vi "Handle Camera Configuration.vi"(9 "CameraNameRef":refnum<vi>, 10 "Camera File Name":string="Camera", 11 "ClusterRef":refnum<vi>) -> ()   [LabVIEW 2016]
uses:
  <vilib>/Rock Robotics/Network Tables/Make Table Operation.ctl
  <vilib>/Utility/config.llb/Read Key (String).vi
  <vilib>/Utility/config.llb/Read Key (I32).vi
  <vilib>/Utility/config.llb/Write Key (String).vi
  <vilib>/Utility/config.llb/Write Key (I32).vi
  <vilib>/Utility/config.llb/NI_LVConfig.lvlib
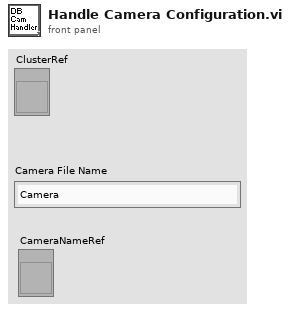
[diagram p1: front panel]
types:
  T1 = typedef "NI_LVConfig.lvlib/Config Data RefNum.ctl" = refnum<k1>
  T2 = cluster{"value":i32, "value":i32, "index":i32, bool}
  T3 = typedef "Make Table Operation.ctl" = enum16{"Get or Add Field", "Get Field or Add Temp", "Replace Temp ID", "Get Field ID - No Add", "Get Table Field IDs", "Get Field ID Info", "Move Field to Temp", "Validate", "Remove Field", "Remove All"}
  T4 = cluster{"Frame Rate":i32, "Compression":i32, "Size":u16, "DB Camera Config":bool}
  T5 = typedef "Field ID.ctl" = i32
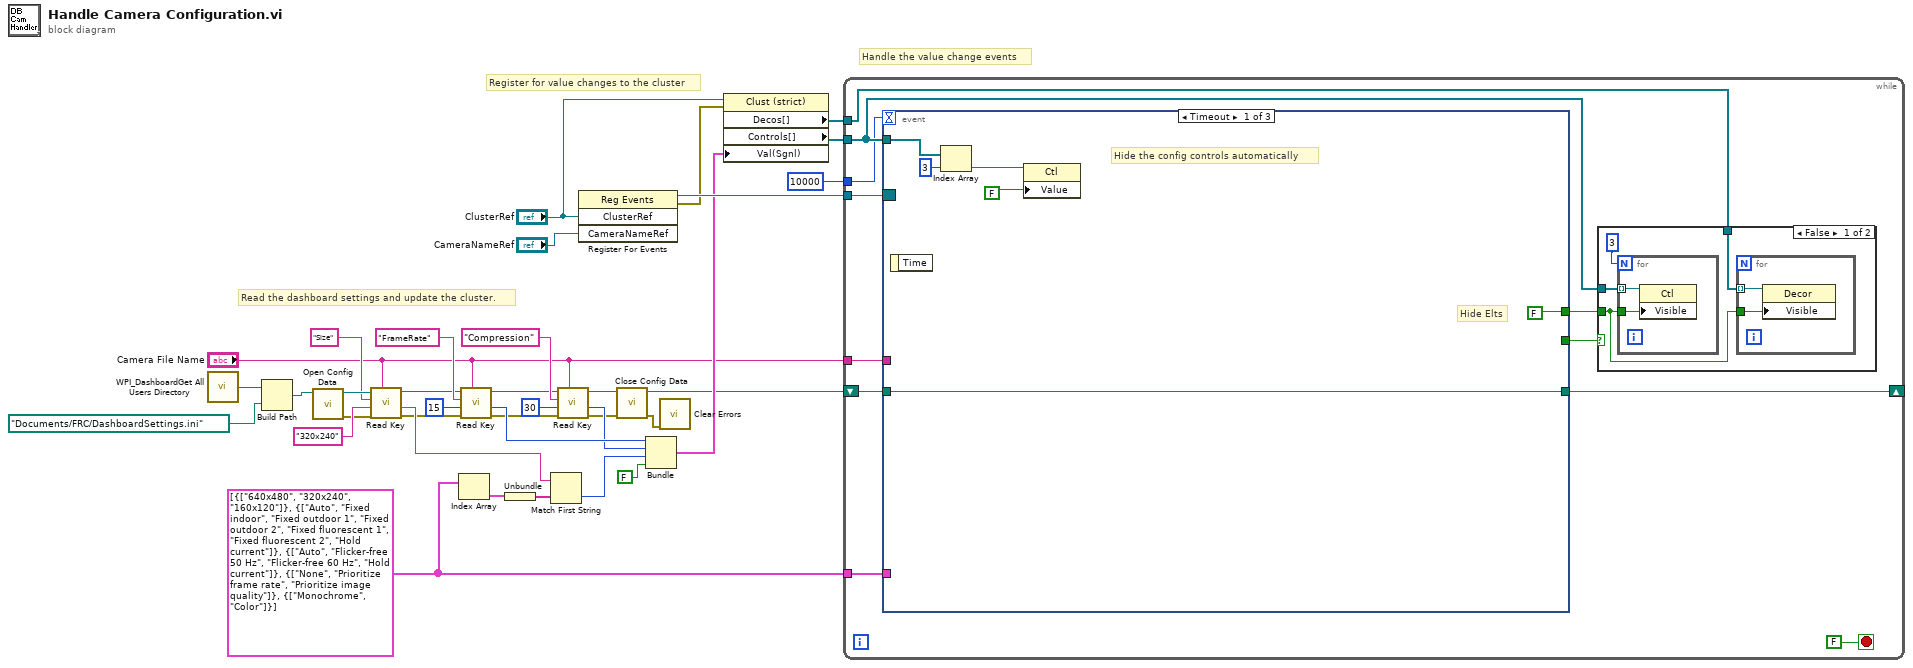
[diagram p0: block diagram]
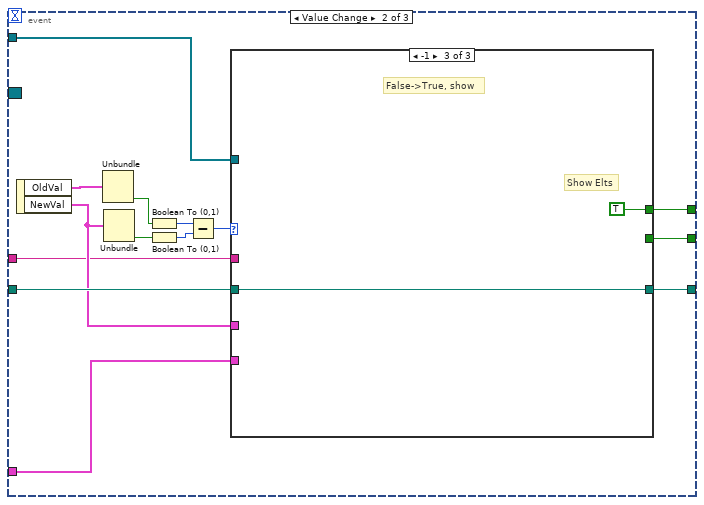
[diagram p3: hidden frame]
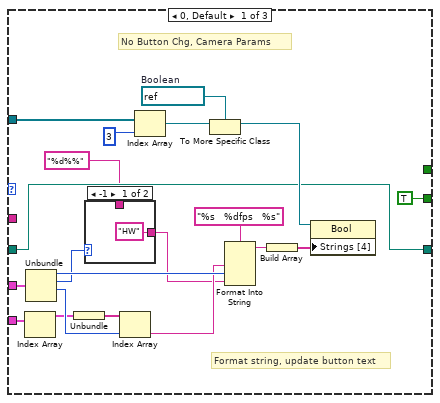
[diagram p4: hidden frame]
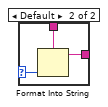
[diagram p5: hidden frame]
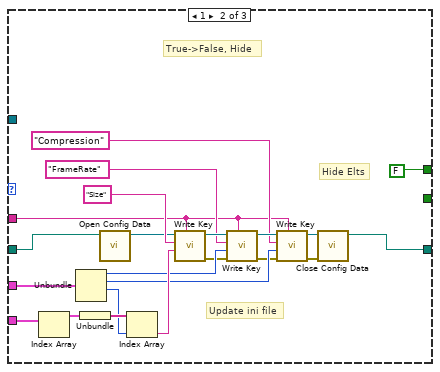
[diagram p6: hidden frame]
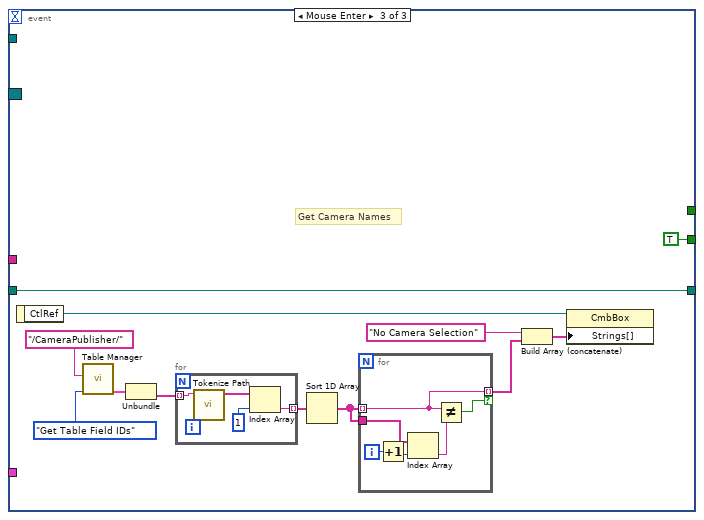
[diagram p7: hidden frame]
diagram:
  w15 = cluster{string[]}[] [{["640x480", "320x240", "160x120"]}, {["Auto", "Fixed indoor", "Fixed outdoor 1", "Fixed outdoor 2", "Fixed fluorescent 1", "Fixed fluorescent 2", "Hold current"]}, {["Auto", "Flicker-free 50 Hz", "Flicker-free 60 Hz", "Hold current"]}, {["None", "Prioritize frame rate", "Prioritize image quality"]}, {["Monochrome", "Color"]}]
  # "Handle the value change events"
  # "Register for value changes to the cluster"
  # "Read the dashboard settings and update the cluster."
  n1 = call <vilib>:"WPI_DashboardGet All Users Directory.vi"() -> ("All User Path"=w33:path)
  n2 = Build Path(base path=w33, name or relative path=path "Documents/FRC/DashboardSettings.ini") -> (appended path=w32:path)
  n3 = call <vilib>:"Open Config Data.vi"("configuration file path"=w32) -> ("error out"=w8:errorcluster, "refnum"=w31:T1)  [unwired: 8 in, 1 out]
  n4 = call-poly <vilib>:"Read Key.vi"("section"="Camera File Name", "error in (no error)"=w8, "default value"="320x240", "key"="Size", "refnum"=w31) -> ("error out"=w7:errorcluster, "value"=w19:string, "refnum out"=w23:T1)  [unwired: 1 in, 3 out]
  n5 = Index Array(array=w15) -> (element=w21:cluster{string[]})  [unwired: 1 in]
  n6 = call-poly <vilib>:"Read Key.vi"("section"="Camera File Name", "error in (no error)"=w7, "default value"=15, "key"="FrameRate", "refnum"=w23) -> ("error out"=w6:errorcluster, "value"=w17:i32, "refnum out"=w22:T1)  [unwired: 4 out]
  n7 = Unbundle(w21) -> (w20:string[])
  n8 = Match First String(2:w20, 3:w19) -> (0:w18:i32)  [unwired: 1 out]
  n9 = call-poly <vilib>:"Read Key.vi"("section"="Camera File Name", "error in (no error)"=w6, "default value"=30, "key"="Compression", "refnum"=w22) -> ("error out"=w3:errorcluster, "value"=w16:i32, "refnum out"=w5:T1)  [unwired: 4 out]
  n10 = register-events("ClusterRef", "CameraNameRef") -> (reference out=w36:refnum<event-registration>, error out=w13:errorcluster)  [unwired: 2 in]
  n11 = call <vilib>:"Close Config Data.vi"("error in (no error)"=w3, "refnum"=w5) -> ("error out"=w2:errorcluster, "file path"=w4:path)  [unwired: 1 in, 7 out]
  n12 = Bundle("value"=w17, "value"=w16, "index"=w18, FALSE) -> (w12:T2)  [unwired: 1 out]
  n13 = call <vilib>:"Clear Errors.vi"("error in (no error)"=w2) -> ()  [unwired: 5 in, 2 out]
  n14 = property class="Clust (strict)"(reference="ClusterRef", error in=w13, "Val(Sgnl)"=w12) -> ("Decos[]"=w10:refnum<vi>[], "Controls[]"=w34:refnum<vi>[])  [unwired: 2 out]
  n15 = while {
    tunnel: w36 -> [w47]
    tunnel: w34 -> [w39]
    shift-right: [w45] -> _
    shift-left: w4 -> [w46]
    tunnel: w15 -> [w44]
    tunnel: "Camera File Name" -> [w42]
    tunnel: w10 -> [w38]
    tunnel: 10000 -> [w37]
    stop <- FALSE stop-if-true
    n16 = event shown="[0] Timeout" {
      selector: w47 -> [_ _ _]
      dyn-events: _ -> [_ _ _]
      timeout: w37 -> [_ _ _]
      tunnel: w46 -> [w60 w69 w133]
      tunnel: [w60 w65 w133] -> w45
      tunnel: w44 -> [_ w67 _]
      tunnel: w39 -> [w59 w66 _]
      tunnel: w42 -> [_ w64 _]
      tunnel: [FALSE w63 _] -> w40
      tunnel: [_ w62 TRUE] -> w41
      event Timeout {
        # "Hide Elts"
        # "Hide the config controls automatically"
        n17 = event-data() -> ()  [unwired: 1 in, 1 out]
        n18 = Index Array(array=w59, index=3) -> (element=w57:refnum<vi>)
        n19 = property class="Ctl"(reference=w57, "Value"=FALSE) -> ()  [unwired: 1 in, 2 out]
      }
      event Value Change {
        n20 = event-data() -> ("OldVal"=w71:T4, "NewVal"=w68:T4)  [unwired: 1 in]
        n21 = Unbundle(w71) -> ("DB Camera Config"=w75:bool)  [unwired: 3 out]
        n22 = Unbundle(w68) -> ("DB Camera Config"=w74:bool)  [unwired: 3 out]
        n23 = Boolean To (0,1)(Boolean=w75) -> (0, 1=w72:i16)
        n24 = Boolean To (0,1)(Boolean=w74) -> (0, 1=w73:i16)
        n25 = Subtract(x=w72, y=w73) -> (x-y=w70:i16)
        n26 = case shown="-1" w70 {
          tunnel: [_ FALSE TRUE] -> w63
          tunnel: [TRUE _ _] -> w62
          tunnel: w69 -> [w79 w102 w122]
          tunnel: w68 -> [w87 w111 _]
          tunnel: w67 -> [w86 w107 _]
          tunnel: w66 -> [w85 _ _]
          tunnel: [w79 w100 w122] -> w65
          tunnel: w64 -> [_ w106 _]
          frame 0, Default {
            w82 = refnum<vi> refnum  # Boolean
            # "Format string, update button text"
            # "No Button Chg, Camera Params"
            n27 = Index Array(array=w86) -> (element=w90:cluster{string[]})  [unwired: 1 in]
            n28 = Unbundle(w87) -> ("Frame Rate"=w94:i32, "Compression"=w76:i32, "Size"=w92:u16)  [unwired: 1 out]
            n29 = Unbundle(w90) -> (w91:string[])
            n30 = case shown="-1" w76 {
              selector: w76 -> [_ w97]
              tunnel: "%d%%" ("format string") -> [_ w99]
              tunnel: ["HW" ("format string") w98] -> w77
              frame -1 {
              }
              frame Default {
                n31 = Format Into String(format string=w99, w97) -> (resulting string=w98:string)  [unwired: 2 in, 1 out]
              }
            }
            n32 = Index Array(array=w91, index=w92) -> (element=w93:string)
            n33 = Index Array(array=w85, index=3) -> (element=w83:refnum<vi>)
            n34 = To More Specific Class(target class=w82, reference=w83) -> (specific class reference=w81:refnum<vi>)  [unwired: 1 in, 1 out]
            n35 = Format Into String(format string="%s   %dfps   %s", w93, w94, w77) -> (resulting string=w89:string)  [unwired: 2 in, 1 out]
            n36 = Build Array(w89) -> (w80:string[])
            n37 = property class="Bool"(reference=w81, "Strings [4]"=w80) -> ()  [unwired: 1 in, 2 out]
          }
          frame 1 {
            # "Update ini file"
            # "Hide Elts"
            # "True->False, Hide"
            n38 = Index Array(array=w107) -> (element=w115:cluster{string[]})  [unwired: 1 in]
            n39 = Unbundle(w111) -> ("Frame Rate"=w110:i32, "Compression"=w109:i32, "Size"=w108:u16)  [unwired: 1 out]
            n40 = Unbundle(w115) -> (w114:string[])
            n41 = call <vilib>:"Open Config Data.vi"("configuration file path"=w102) -> ("refnum"=w101:T1)  [unwired: 8 in, 2 out]
            n42 = Index Array(array=w114, index=w108) -> (element=w113:string)
            n43 = call-poly <vilib>:"Write Key.vi"("section"=w106, "value"=w113, "key"="Size", "refnum"=w101) -> ("error out"=w105:errorcluster, "refnum out"=w120:T1)  [unwired: 2 in, 4 out]
            n44 = call-poly <vilib>:"Write Key.vi"("section"=w106, "error in (no error)"=w105, "value"=w110, "key"="FrameRate", "refnum"=w120) -> ("error out"=w104:errorcluster, "refnum out"=w119:T1)  [unwired: 5 out]
            n45 = call-poly <vilib>:"Write Key.vi"("section"=w106, "error in (no error)"=w104, "value"=w109, "key"="Compression", "refnum"=w119) -> ("error out"=w103:errorcluster, "refnum out"=w112:T1)  [unwired: 5 out]
            n46 = call <vilib>:"Close Config Data.vi"("error in (no error)"=w103, "refnum"=w112) -> ("file path"=w100:path)  [unwired: 1 in, 8 out]
          }
          frame -1 {
            # "Show Elts"
            # "False->True, show"
          }
        }
      }
      event Mouse Enter {
        # "Get Camera Names"
        n47 = event-data() -> ("CtlRef"=w135:refnum<vi>)  [unwired: 1 in]
        n48 = call <vilib>:"Table Manager.vi"("Operation"=Make_Table_Operation."Get Table Field IDs", "Entry Name"="/CameraPublisher/") -> ("Entries"=w130:cluster{"Entry IDs":T5[], "Names":string[]})  [unwired: 6 in, 3 out]
        n49 = Unbundle(w130) -> ("Names"=w127:string[])  [unwired: 1 out]
        n50 = for {
          tunnel: w127 -> [w145] mode=indexing
          tunnel: [w142] -> w126 mode=indexing
          n51 = call <vilib>:"Tokenize Path.vi"("Name"=w145) -> ("Array"=w144:string[])  [unwired: 10 in]
          n52 = Index Array(array=w144, index=1) -> (element=w142:string)
        }
        n53 = Sort 1D Array(array=w126) -> (sorted array=w125:string[])
        n54 = for {
          tunnel: w125 -> [w137] mode=indexing
          tunnel: w125 -> [w139]
          tunnel: [w137] -> w124 mode=indexing if=w136
          i -> [w141]
          n55 = Increment(x=w141) -> (x+1=w140:i32)
          n56 = Index Array(array=w139, index=w140) -> (element=w138:string)
          n57 = Not Equal?(x=w137, y=w138) -> (x != y?=w136:bool)
        }
        n58 = Build Array (concatenate)("No Camera Selection", w124) -> (w128:string[])
        n59 = property class="CmbBox"(reference=w135, "Strings[]"=w128) -> ()  [unwired: 1 in, 2 out]
      }
    }
    n60 = case shown="False" w41 {
      tunnel: w39 -> [w51 _]
      tunnel: w40 -> [w48 _]
      tunnel: w38 -> [w49 _]
      frame False {
        n61 = for {
          N: 3 -> [_]
          tunnel: w51 -> [w55] mode=indexing
          tunnel: w48 -> [w54]
          n62 = property class="Ctl"(reference=w55, "Visible"=w54) -> ()  [unwired: 1 in, 2 out]
        }
        n63 = for {
          tunnel: w49 -> [w53] mode=indexing
          tunnel: w48 -> [w52]
          n64 = property class="Decor"(reference=w53, "Visible"=w52) -> ()  [unwired: 1 in, 2 out]
        }
      }
      frame True {
      }
    }
  }
